vi "FGV_Settings IO Rule.vi"(7 "Command_Settings IO Rule":T1(ring), 8 "Error In":errorcluster, 11 "Settings Type IN":string) -> (0 "Error Out":errorcluster, 2 "Specified Settings (OUT)":string[](array[string]), 3 "Settings Table (OUT)":string[][](array[string]))   [LabVIEW 2012]
doc: "SciScan 1.2 160622"
uses:
  <vilib>/Utility/file.llb/Read From Spreadsheet File (string).vi
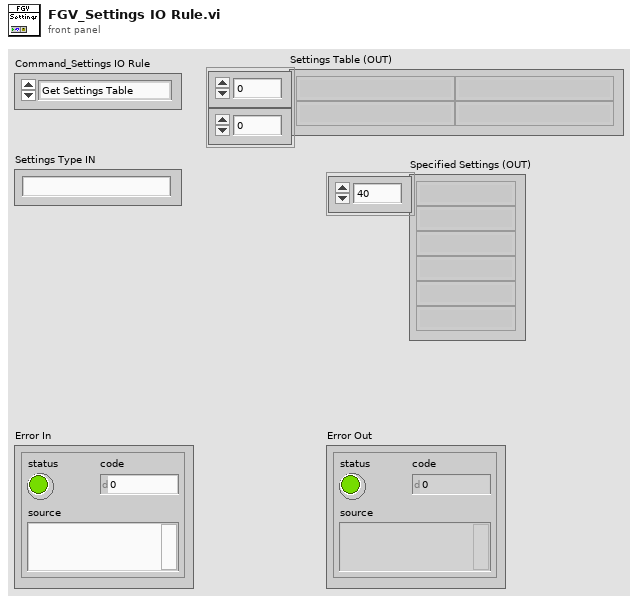
[diagram p1: front panel]
types:
  T1 = enum16{"Get Settings Table ", "Read Settings File", "Get Specified Settings"}
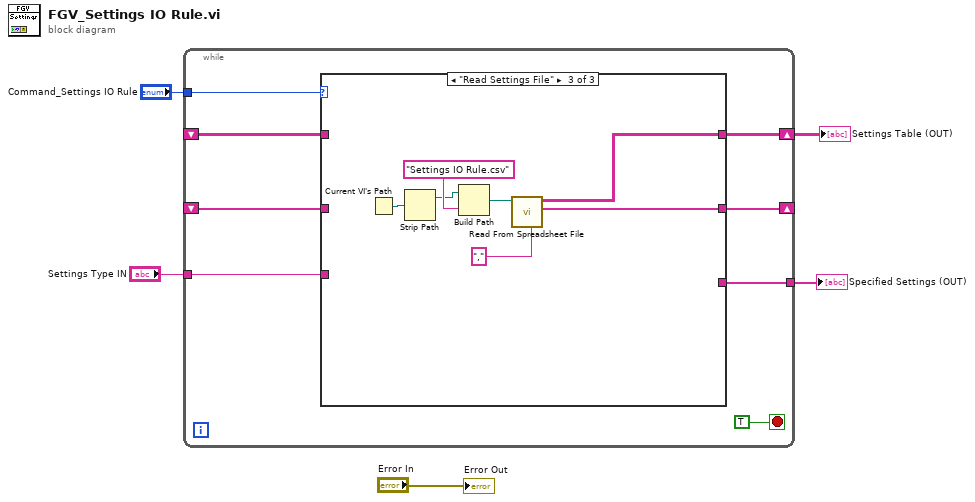
[diagram p0: block diagram]
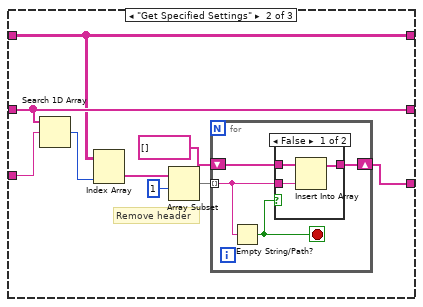
[diagram p3: hidden frame]
diagram:
  n1 = while {
    tunnel: "Command_Settings IO Rule" -> [w12]
    shift-right: [w11] -> w4
    shift-left: _ -> [w9]
    shift-right: [w10] -> _
    shift-left: _ -> [w8]
    tunnel: "Settings Type IN" -> [w7]
    tunnel: [w6] -> w2
    stop <- TRUE stop-if-true
    n2 = case shown="\"Read Settings File\"" w12 {
      tunnel: [w15 w22 w37] -> w11
      tunnel: [w14 w24 w36] -> w10
      tunnel: w9 -> [w15 w22 _]
      tunnel: w8 -> [w14 w24 _]
      tunnel: w7 -> [_ w23 _]
      tunnel: [_ w18 _] -> w6
      frame "Get Settings Table ", Default {
      }
      frame "Get Specified Settings" {
        # "Remove header"
        n3 = Search 1D Array(1D array=w24, element=w23) -> (index of element=w21:i32)  [unwired: 1 in]
        n4 = Index Array(array=w22, index (col)=w21) -> (element=w20:string[])  [unwired: 1 in]
        n5 = Array Subset(array=w20, index=1) -> (w19:string[])  [unwired: 1 in]
        n6 = for {
          tunnel: w19 -> [w27] mode=indexing
          shift-right: [w26] -> w18
          shift-left: string[] [] -> [w25]
          stop <- w28 stop-if-true
          n7 = Empty String/Path?(string/path=w27) -> (empty?=w28:bool)
          n8 = case shown="False" w28 {
            tunnel: w27 -> [w29 _]
            tunnel: [w31 w32] -> w26
            tunnel: w25 -> [w30 w32]
            frame False {
              n9 = Insert Into Array(array=w30, new element=w29) -> (w31:string[])  [unwired: 1 in]
            }
            frame True {
            }
          }
        }
      }
      frame "Read Settings File" {
        n10 = Current VI's Path() -> (path=w34:path)
        n11 = Strip Path(path=w34) -> (stripped path=w33:path)  [unwired: 1 out]
        n12 = Build Path(base path=w33, name or relative path="Settings IO Rule.csv") -> (appended path=w38:path)
        n13 = call-poly <vilib>:"Read From Spreadsheet File.vi"("delimiter (\\t)"="," ("delimiter (\\t)"), "file path (dialog if empty)"=w38) -> ("first row"=w36:string[], "all rows"=w37:string[][])  [unwired: 5 in, 3 out]
      }
    }
  }
  "Settings Table (OUT)" <- w4
  "Specified Settings (OUT)" <- w2
  "Error Out" <- "Error In"
